vi "String.vi"(8 "Error In":errorcluster) -> (0 "Error Out":errorcluster)   [LabVIEW 2017, in "Tests.lvlib" / "Status.lvlib"]
uses:
  Status.lvlib
  src/LabPack/Public/Controls/Status.ctl
  <vilib>/addons/_JKI Toolkits/Caraya/classes/Test/Test.lvclass
  src/LabPack/LabPack.lvlib
  <vilib>/addons/_JKI Toolkits/Caraya/classes/Assert/Assert.lvclass
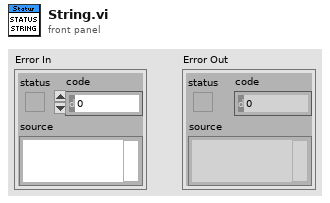
[diagram p1: front panel]
types:
  T1 = typedef "LabPack.lvlib/Status.ctl" = enum32{"OK", "Out of Memory", "Null Value", "Encoder"}
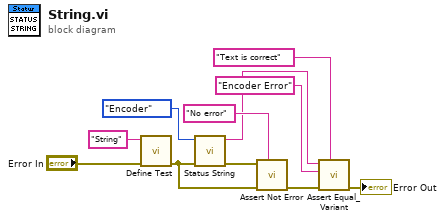
[diagram p0: block diagram]
diagram:
  n1 = call <vilib>:"Define Test.vi"("error in (no error)"="Error In", "Label (VI Title)"="String") -> ("error out"=w6:errorcluster)  [unwired: 9 in]
  n2 = call "Status String.vi"("Error In"=w6, "Status"=Status."Encoder") -> ("Error Out"=w8:errorcluster, "Text"=w3:string)  [unwired: 8 in]
  n3 = call <vilib>:"Assert Not Error.vi"("Label"="No error", "error in (no error)"=w6, "Not Error?"=w8) -> ("error out"=w5:errorcluster)  [unwired: 8 in]
  n4 = call <vilib>:"Assert Equal_Variant.vi"("Label"="Text is correct", "error in (no error)"=w5, "Y"="Encoder Error" ("Text"), "X"=w3) -> ("error out"=→"Error Out":errorcluster)  [unwired: 7 in]
